vi "ex6_trigger.vi"() -> ()   [LabVIEW 2012]
uses:
  \\csehomes\csehome$/dsp15/My Documents/Mini-Cryo Automation Software/Patiwet/QCam.llb/QCam Grab Abort.vi
panel:
  in  "Halt loop":bool
  in  "Trigger Mode":T1(ring)=enum."Edge hi"
  in  "stop":bool
  out "error status":errorcluster
  out "Preview Window":picture
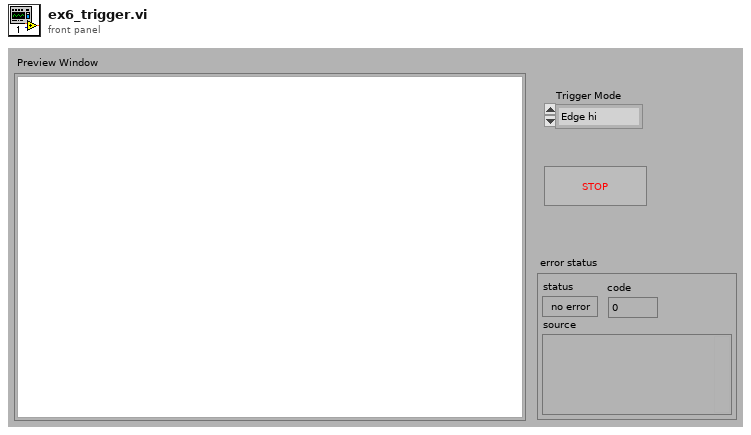
[diagram p1: front panel]
types:
  T1 = enum32{"Freerun", "Edge hi", "Edge low", "Pulse hi", "Pulse low", "Software"}
  T2 = typedef "IMAQ Image.ctl" = refnum<image>
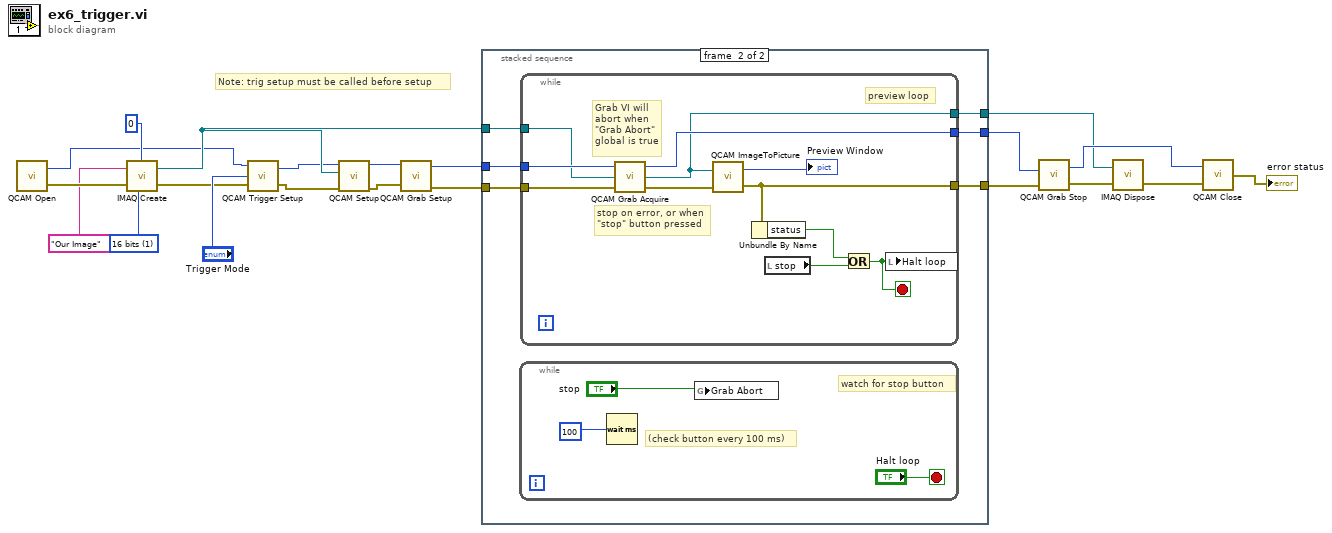
[diagram p0: block diagram]
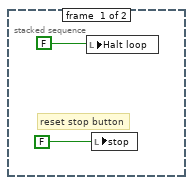
[diagram p2: hidden frame]
diagram:
  w20 = u32 1 items=["8 bits", "16 bits"] ("Image Type")
  # "Note: trig setup must be called before setup"
  n1 = call "QCAM Open.vi"() -> ("error out"=w21:errorcluster, "cameraId out"=w1:u32)  [unwired: 2 in]
  n2 = call "IMAQ Create"("Border Size"=0, "Image Name"="Our Image", "Image Type"=w20, "error in (no error)"=w21) -> ("New Image"=w14:T2, "error out"=w4:errorcluster)  [unwired: 1 out]
  n3 = call "QCAM Trigger Setup.vi"("error in (no error)"=w4, "trigger mode"="Trigger Mode", "camera Id"=w1) -> ("error out"=w3:errorcluster, "camera Id out"=w2:u32)
  n4 = call "QCAM Setup.vi"("error in (no error)"=w3, "Image"=w14, "cameraId"=w2) -> ("error out"=w6:errorcluster, "cameraId out"=w5:u32)  [unwired: 3 in, 4 out]
  n5 = call "QCAM Grab Setup.vi"("error in (no error)"=w6, "cameraId"=w5) -> ("error out"=w16:errorcluster, "cameraId out"=w15:u32)
  n6 = stacked-sequence {
    tunnel: w16 -> [_ w29]
    tunnel: w15 -> [_ w28]
    tunnel: w14 -> [_ w27]
    tunnel: [_ w26] -> w13
    tunnel: [_ w25] -> w12
    tunnel: [_ w24] -> w9
    frame #0 {
      # "reset stop button"
      n7 = local write "Halt loop"(FALSE) -> ()
      n8 = local write "stop"(FALSE) -> ()
    }
    frame #1 {
      n9 = while {
        stop <- "Halt loop" stop-if-true
        # "(check button every 100 ms)"
        # "watch for stop button"
        n10 = Wait (ms)(milliseconds to wait=100) -> ()  [unwired: 1 out]
        n11 = global write "QCam Grab Abort.vi" "Grab Abort"("stop") -> ()
      }
      n12 = while {
        tunnel: [w35] -> w24
        tunnel: [w32] -> w26
        tunnel: w27 -> [w33]
        tunnel: w28 -> [w34]
        tunnel: w29 -> [w37]
        tunnel: [w38] -> w25
        stop <- w30 stop-if-true
        # "Grab VI will abort when \"Grab Abort\" global is true"
        # "preview loop"
        # "stop on error, or when \"stop\" button pressed"
        n13 = call "QCAM Grab Acquire.vi"("error in (no error)"=w37, "Image"=w33, "cameraId"=w34) -> ("error out"=w39:errorcluster, "Image Out"=w35:T2, "cameraId out"=w38:u32)
        n14 = call <userlib>:"QCAM ImageToPicture.vi"("error in (no error)"=w39, "Image"=w35) -> ("error out"=w32:errorcluster, "Picture Out"=→"Preview Window":picture)
        n15 = Unbundle By Name(w32) -> ("status"=w36:bool)
        n16 = local read "stop"() -> (w31:bool)
        n17 = Or(x=w36, y=w31) -> (x .or. y?=w30:bool)
        n18 = local write "Halt loop"(w30) -> ()
      }
    }
  }
  n19 = call "QCAM Grab Stop.vi"("error in (no error)"=w13, "cameraId"=w12) -> ("error out"=w19:errorcluster, "cameraId Out"=w17:u32)
  n20 = call "IMAQ Dispose"("Image"=w9, "error in (no error)"=w19) -> ("error out"=w18:errorcluster)  [unwired: 1 in, 3 out]
  n21 = call "QCAM Close.vi"("error in (no error)"=w18, "cameraId"=w17) -> ("error out"=→"error status":errorcluster)
